vi "STS_Get_Meas_Monitor_Rawdata.vi"(8 "错误输入（无错误）":errorcluster, 10 "setting":refnum<k24>, 11 ".NET引用句柄输入":refnum<k24>) -> (0 "error out":errorcluster, 1 "monitordata":sgl[](array[numeric]), 3 "引用输出":refnum<k24>)   [LabVIEW 2017]
doc: "monitor data is 1 data for each sweep. It can be overwrite."
uses:
  D:/test/ILSTS/LV_IL/LV_IL_Sample_x86/DLL/STSProcess.dll
  DLL/STSProcess.dll
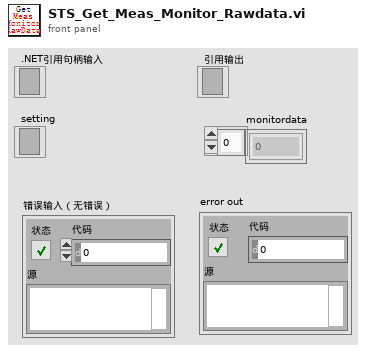
[diagram p1: front panel]
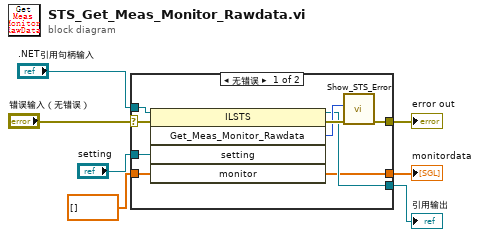
[diagram p0: block diagram]
diagram:
  n1 = case shown="无错误" "错误输入（无错误）" {
    selector: "错误输入（无错误）" -> [w15 w19]
    tunnel: ".NET引用句柄输入" -> [w16 w18]
    tunnel: [w12 w19] -> w5
    tunnel: [w11 w18] -> w4
    tunnel: sgl[] [] ("powerdata") -> [w10 w17]
    tunnel: [w9 w17] -> w2
    tunnel: "setting" -> [w8 _]
    frame No Error {
      n2 = invoke class="ILSTS" method="Get_Meas_Monitor_Rawdata"(reference=w16, error in=w15, "setting"=w8, "monitor"=w10) -> (reference out=w11:refnum<k24>, error out=w14:errorcluster, "Get_Meas_Monitor_Rawdata"=w13:i32, "monitor"=w9:sgl[])  [unwired: 1 in, 1 out]
      n3 = call "Show_STS_Error.vi"("error in (no error)"=w14, "Error"=w13) -> ("error out"=w12:errorcluster)  [unwired: 9 in]
    }
    frame Error {
    }
  }
  "error out" <- w5
  "引用输出" <- w4
  "monitordata" <- w2
